vi "PropPage_Pos&Size.vi"() -> (2 "OKtoQuit":bool)   [LabVIEW 2011]
doc: "Property Page plugin template.\n\n\nGeorge Zou\nhttp://webspace.webring.com/people/og/gtoolbox\n\n2016.7"
panel:
  in  "height":i32 caption="Height" step=1
  in  "width":i32 caption="Width" step=1
  in  "QueueName":string
  in  "Main Ref Array In":refnum<vi>[](array[refnum])
  in  "top":i32 caption="Top" step=1
  in  "left":i32 caption="Left" step=1
  in  "close":bool caption="Close"
  # "Position"
  # "Do not change.  Input/output used by the caller."
  # "Take a look PropPage_TabularAppearance.vi.  Max FP to see input/output."
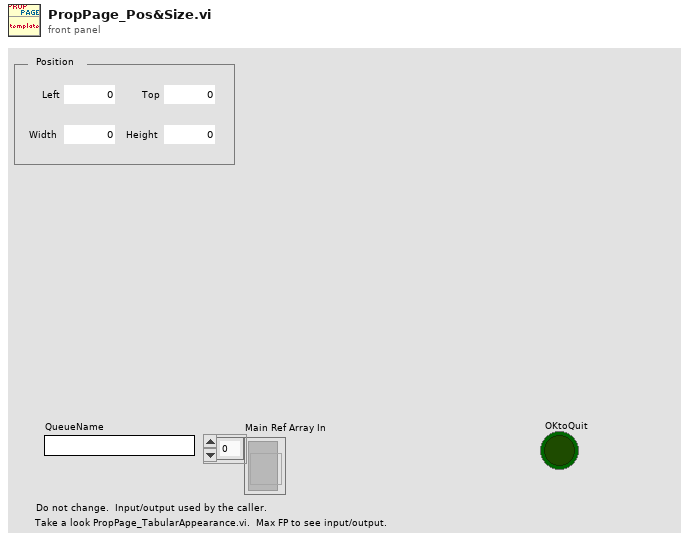
[diagram p1: front panel]
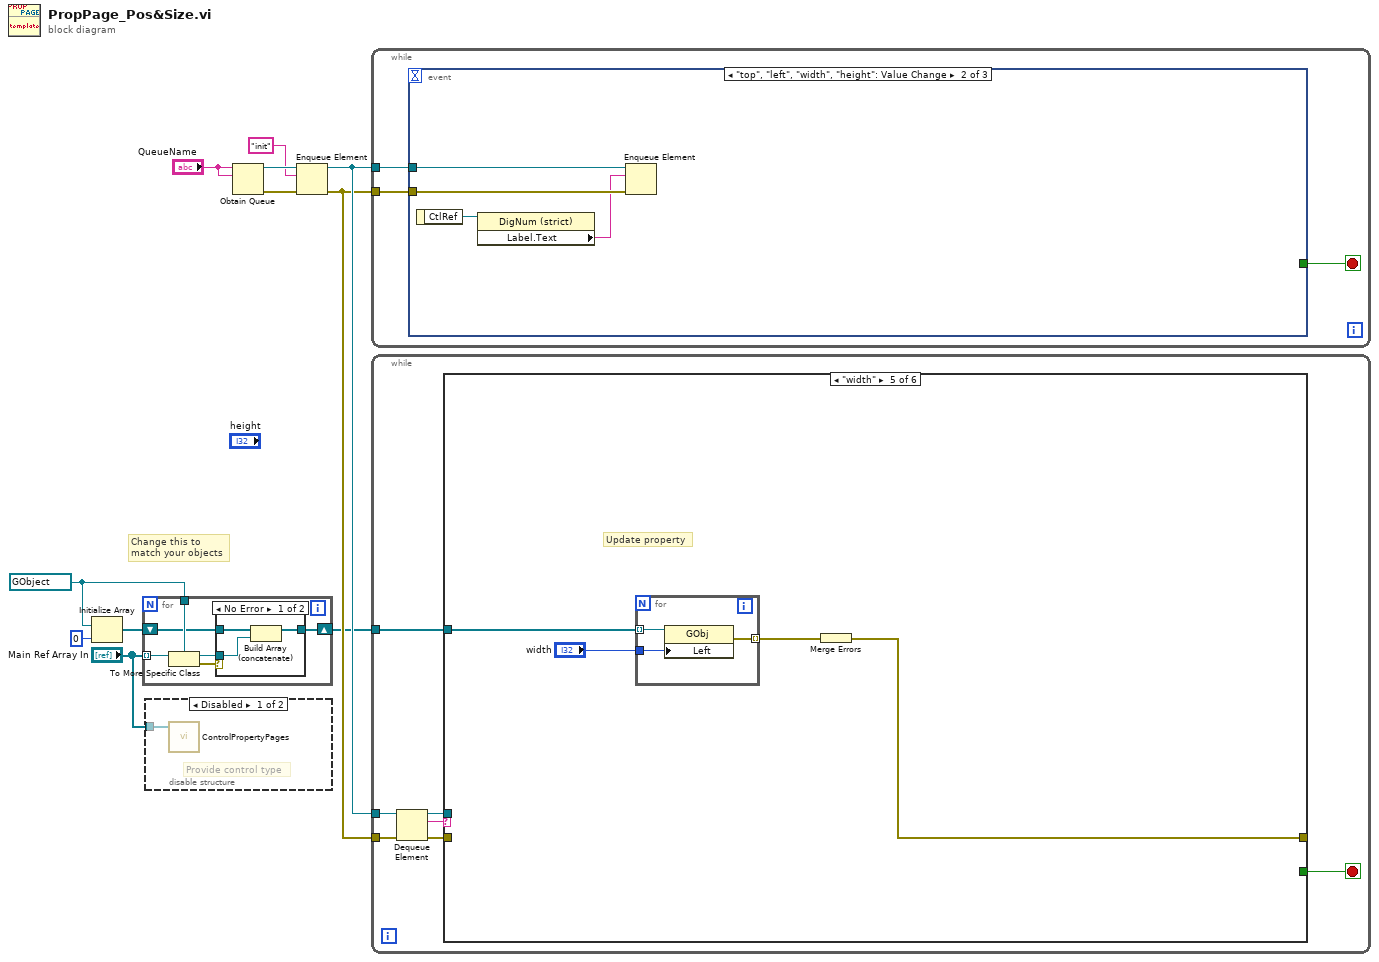
[diagram p0: block diagram]
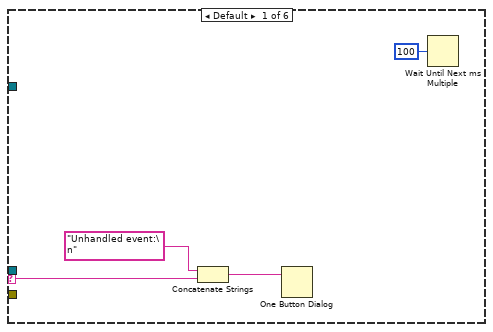
[diagram p4: hidden frame]
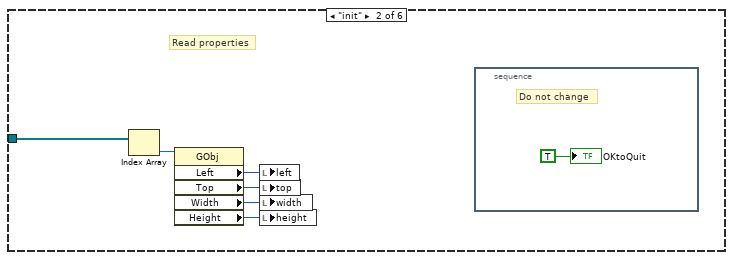
[diagram p5: hidden frame]
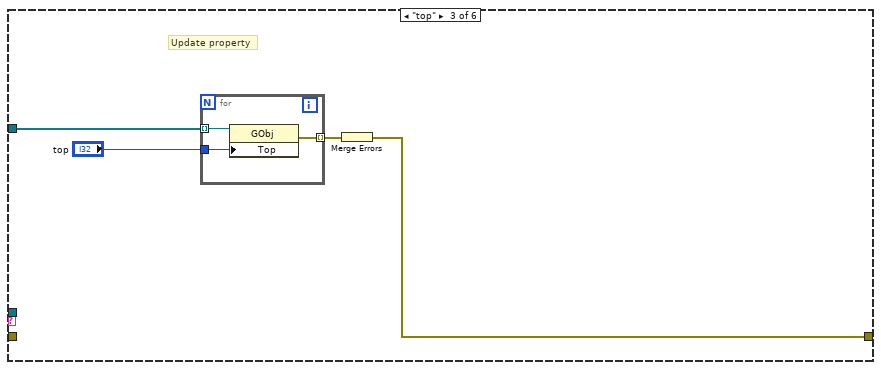
[diagram p6: hidden frame]
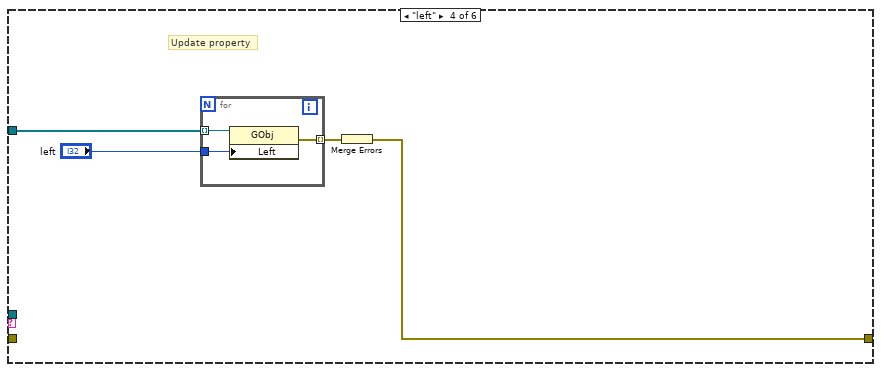
[diagram p7: hidden frame]
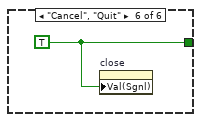
[diagram p8: hidden frame]
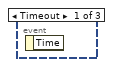
[diagram p9: hidden frame]
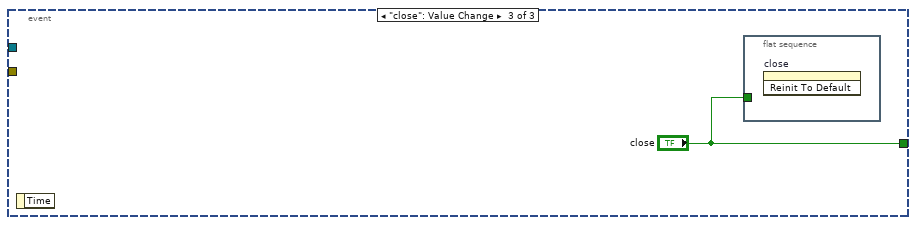
[diagram p10: hidden frame]
diagram:
  w3 = refnum<vi> refnum ("GObj Refnum")
  # "Change this to match your objects"
  n1 = Initialize Array(w3, 0 ("dimension size")) -> (w1:refnum<vi>[])
  n2 = for {
    tunnel: "Main Ref Array In" -> [w17] mode=indexing
    tunnel: w3 -> [w15]
    shift-right: [w13] -> w7
    shift-left: w1 -> [w14]
    n3 = To More Specific Class(target class=w15, reference=w17) -> (specific class reference=w16:refnum<vi>, error out=w12:errorcluster)  [unwired: 1 in]
    n4 = case shown="No Error" w12 {
      tunnel: w14 -> [w19 w21]
      tunnel: w16 -> [w18 _]
      tunnel: [w20 w21] -> w13
      frame No Error {
        n5 = Build Array (concatenate)(w19, w18) -> (w20:refnum<vi>[])
      }
      frame Error {
      }
    }
  }
  n6 = disable-structure shown="Disabled" {
    disable-tunnel: "Main Ref Array In" -> [w22 _]
    frame Disabled {
      # "Provide control type"
      n7 = call "ControlPropertyPages.vi"("Num Refnum Array"=w22) -> ()  [unwired: 2 in, 1 out]
    }
    frame Enabled {
    }
  }
  n8 = Obtain Queue(name (unnamed)="QueueName", element data type="QueueName") -> (queue out=w8:refnum<queue>, error out=w9:errorcluster)  [unwired: 3 in, 1 out]
  n9 = Enqueue Element(queue=w8, element="init" ("event"), error in (no error)=w9) -> (queue out=w11:refnum<queue>, error out=w10:errorcluster)  [unwired: 1 in, 1 out]
  n10 = while {
    tunnel: w11 -> [w25]
    tunnel: w10 -> [w24]
    stop <- w23 stop-if-true
    n11 = event shown="[1] \"top\", \"left\", \"width\", \"height\": Value Change" {
      selector: _ -> [_ _ _]
      dyn-events: _ -> [_ _ _]
      timeout: _ -> [_ _ _]
      tunnel: w25 -> [_ w29 _]
      tunnel: w24 -> [_ w28 _]
      tunnel: [_ _ "close"] -> w23
      event Timeout {
        n12 = event-data() -> ()  [unwired: 1 in, 1 out]
      }
      event "top", "left", "width", "height": Value Change {
        n13 = event-data() -> ("CtlRef"=w27:refnum<vi>)  [unwired: 1 in]
        n14 = property class="DigNum (strict)"(reference=w27) -> ("Label.Text"=w26:string)  [unwired: 1 in, 2 out]
        n15 = Enqueue Element(queue=w29, element=w26, error in (no error)=w28) -> ()  [unwired: 1 in, 3 out]
      }
      event "close": Value Change {
        n16 = event-data() -> ()  [unwired: 1 in, 1 out]
        n17 = flat-sequence {
          tunnel: "close" -> [_]
          frame #0 {
            n18 = invoke on="close" class="Bool (strict)" method="Reinit To Default"() -> ()  [unwired: 3 in, 3 out]
          }
        }
      }
    }
  }
  n19 = while {
    tunnel: w10 -> [w37]
    tunnel: w11 -> [w36]
    tunnel: w7 -> [w32]
    stop <- w34 stop-if-true
    n20 = Dequeue Element(queue=w36, error in (no error)=w37) -> (queue out=w33:refnum<queue>, element=w31:string, error out=w35:errorcluster)  [unwired: 1 in, 1 out]
    n21 = case shown="\"width\"" w31 {
      selector: w31 -> [w41 _ _ _ _ _]
      tunnel: w35 -> [_ _ _ _ _ _]
      tunnel: [_ _ _ _ _ w70] -> w34
      tunnel: w33 -> [_ _ _ _ _ _]
      tunnel: w32 -> [_ w47 w52 w59 w66 _]
      tunnel: [_ _ w50 w57 w63 _] -> _
      frame Default {
        n22 = Concatenate Strings("Unhandled event:\n" ("string"), w41) -> (w40:string)
        n23 = One Button Dialog(message=w40) -> ()  [unwired: 1 in, 1 out]
        n24 = Wait Until Next ms Multiple(millisecond multiple=u32 100) -> ()  [unwired: 1 out]
      }
      frame "init" {
        # "Read properties"
        n25 = Index Array(array=w47) -> (element=w46:refnum<vi>)  [unwired: 1 in]
        n26 = property class="GObj"(reference=w46) -> ("Left"=w45:i32, "Top"=w44:i32, "Width"=w43:u32, "Height"=w42:u32)  [unwired: 1 in, 2 out]
        n27 = local write "left"(w45) -> ()
        n28 = local write "top"(w44) -> ()
        n29 = local write "width"(w43) -> ()
        n30 = local write "height"(w42) -> ()
        n31 = stacked-sequence {
          frame #0 {
            # "Do not change"
            "OKtoQuit" <- TRUE ("OKtoQuit")
          }
        }
      }
      frame "top" {
        # "Update property"
        n32 = for {
          tunnel: w52 -> [w55] mode=indexing
          tunnel: "top" -> [w54]
          tunnel: [w53] -> w51 mode=indexing
          n33 = property class="GObj"(reference=w55, "Top"=w54) -> (error out=w53:errorcluster)  [unwired: 1 in, 1 out]
        }
        n34 = Merge Errors(w51) -> (w50:errorcluster)
      }
      frame "left" {
        # "Update property"
        n35 = for {
          tunnel: w59 -> [w62] mode=indexing
          tunnel: "left" -> [w61]
          tunnel: [w60] -> w58 mode=indexing
          n36 = property class="GObj"(reference=w62, "Left"=w61) -> (error out=w60:errorcluster)  [unwired: 1 in, 1 out]
        }
        n37 = Merge Errors(w58) -> (w57:errorcluster)
      }
      frame "width" {
        # "Update property"
        n38 = for {
          tunnel: w66 -> [w67] mode=indexing
          tunnel: "width" -> [w69]
          tunnel: [w68] -> w64 mode=indexing
          n39 = property class="GObj"(reference=w67, "Left"=w69) -> (error out=w68:errorcluster)  [unwired: 1 in, 1 out]
        }
        n40 = Merge Errors(w64) -> (w63:errorcluster)
      }
      frame "Cancel", "Quit" {
        w70 = TRUE
        n41 = property on="close" class="Bool (strict)"("Val(Sgnl)"=w70) -> ()  [unwired: 2 in, 2 out]
      }
    }
  }
